vi "Conversão Pressão.vi"(1 "MIN":i32=-50, 2 "MAX":i32=50, 3 "input":dbl[](array[numeric])) -> (0 "output":dbl[](array[numeric]))   [LabVIEW 2019]
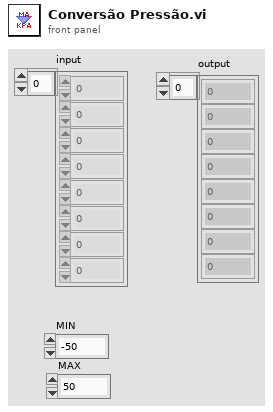
[diagram p1: front panel]
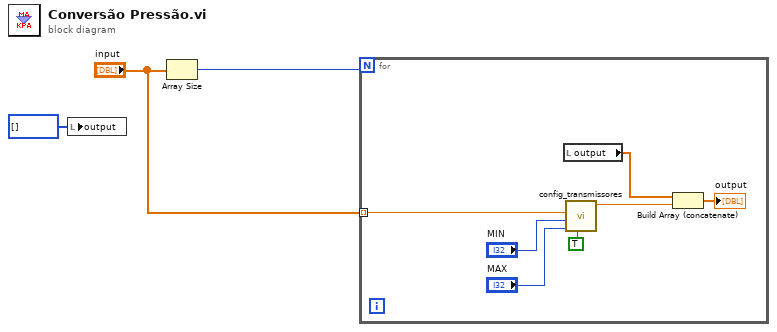
[diagram p0: block diagram]
diagram:
  n1 = local write "output"(i32[] [] ("output")) -> ()
  n2 = Array Size(array="input") -> (size(s)=w3:i32)
  n3 = for {
    N: w3 -> [_]
    tunnel: "input" -> [w7] mode=indexing
    n4 = local read "output"() -> (w4:dbl[])
    n5 = call "config_transmissores.vi"("conversao corrente"=TRUE, "MAX"="MAX", "MIN"="MIN", "Corrente(mA)"=w7) -> ("valor"=w5:dbl)  [unwired: 7 in]
    n6 = Build Array (concatenate)(w4, w5) -> (→"output":dbl[])
  }
